vi "Power Qualtiy - 2.vi"() -> ()   [LabVIEW 2015]
uses:
  <vilib>/addons/Electrical Power/PQ/Common/Controls/ep_AI Data Channel.ctl
  <vilib>/addons/Electrical Power/PQ/Common/Controls/ep_Wiring.ctl
  <vilib>/addons/Electrical Power/PQ/Utility/Initialize System (Single Line).vi
  <vilib>/addons/Electrical Power/Basic/Measurement/RMS (1 Channel).vi
  <vilib>/express/express analysis/Spectral/Block/exnSpectralBlock spectral measurements RMS poly.vi
  <vilib>/express/express analysis/Spectral/Block/exnSpectralBlock spectral measurements RMS DDT.vi
  <vilib>/express/express analysis/Spectral/XNode/ExpressSpectralMeasurementsBlockNode.xnode
  <vilib>/addons/Electrical Power/PQ/NI_EP_Power Quality.lvlib
  <vilib>/addons/Electrical Power/Basic/NI_EP_Basic.lvlib
panel:
  out "Waveform Graph 2":dynamicdata(graph)
  out "THD [%]":dbl[](array[numeric])
  out "RMS value":dbl
  out "Waveform Graph":dynamicdata(graph)
  out "spectra":T2(array[cluster])
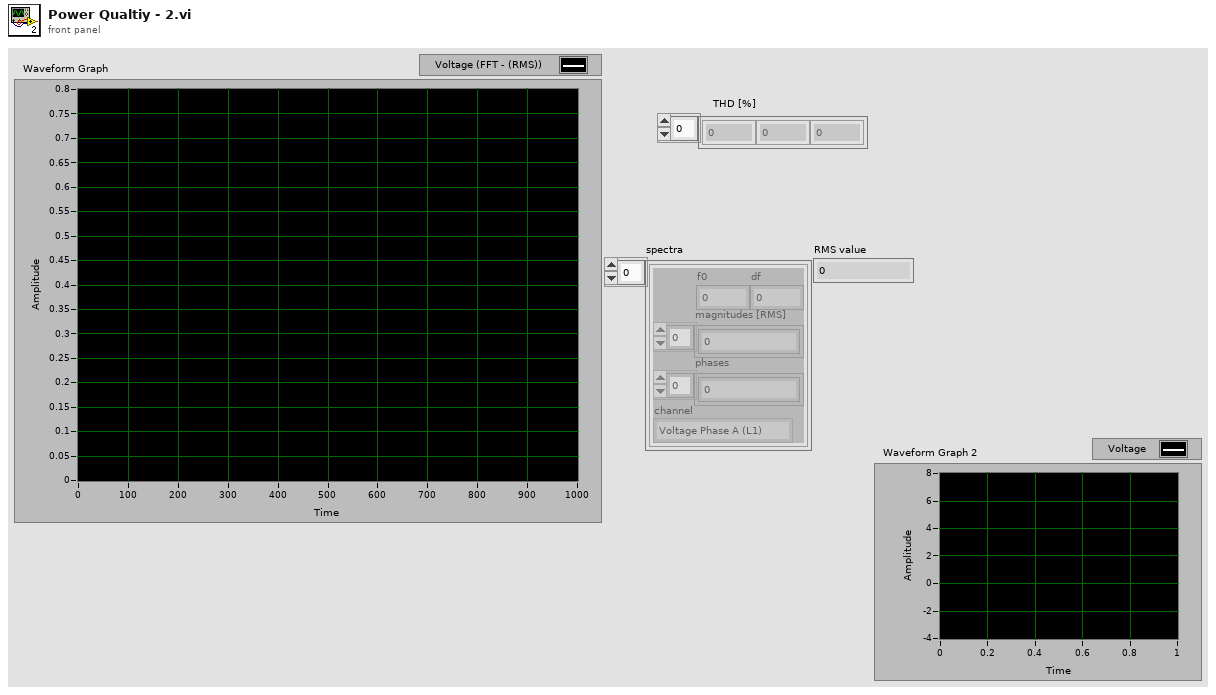
[diagram p1: front panel]
types:
  T1 = typedef "NI_EP_Power Quality.lvlib/ep_AI Data Channel.ctl" = enum16{"Voltage Phase A (L1)", "Voltage Phase B (L2)", "Voltage Phase C (L3)", "Voltage Phase N (Neutral)", "Current Phase A (L1)", "Current Phase B (L2)", "Current Phase C (L3)", "Current Phase N (Neutral)"}
  T2 = cluster{"f0":dbl, "df":dbl, "magnitudes [RMS]":dbl[], "phases":dbl[], "channel":T1}[]
  T3 = typedef "NI_EP_Power Quality.lvlib/ep_Wiring.ctl" = enum16{"4xUph + 4xI", "3xUph + 4xI", "3xUline + 4xI", "3xUph + 3xI", "3xUline + 3xI", "3xUph + 2xI", "3xUline + 2xI", "1xUph + 1xI"}
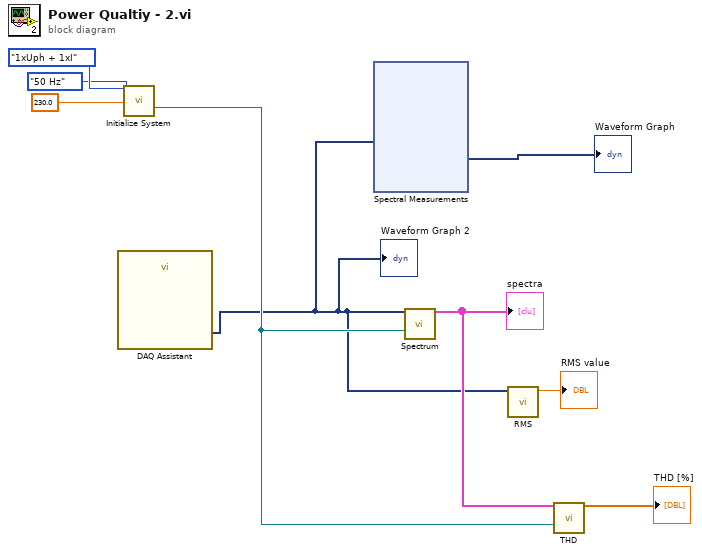
[diagram p0: block diagram]
diagram:
  n1 = call "DAQ Assistant"() -> ("data"=w1:dynamicdata)  [unwired: 17 in, 2 out]
  "Waveform Graph 2" <- w1
  n2 = call-poly <vilib>:"Initialize System.vi"("wiring"=ep_Wiring."1xUph + 1xI", "nominal frequency"=enum16{"50 Hz", "60 Hz"}."50 Hz", "nominal voltage (230 V)"=230.0) -> ("system info out"=w4:refnum<class "EP System Info.lvclass">)  [unwired: 10 in, 2 out]
  n3 = xnode "Spectral Measurements"("Signals"=w1) -> ("FFT - (RMS)"=→"Waveform Graph":dynamicdata)  [unwired: 1 in, 2 out]
  n4 = call <vilib>:"Spectrum.vi"("waveforms"=w1, "system info in"=w4) -> ("spectra"=w3:T2)  [unwired: 11 in, 2 out]
  "spectra" <- w3
  n5 = call-poly <vilib>:"RMS.vi"("waveform"=w1) -> ("RMS value"=→"RMS value":dbl)  [unwired: 9 in, 1 out]
  n6 = call <vilib>:"THD.vi"("spectra"=w3, "system info in"=w4) -> ("THD [%]"=→"THD [%]":dbl[])  [unwired: 11 in, 2 out]
